vi "Read CorrectionFactors.vi"(8 "error in (no error)":errorcluster, 11 "SamplerPluginsBase in":refnum<class "SamplerPluginsBase.lvclass">) -> (0 "error out":errorcluster, 2 "CorrectionFactors":T1, 3 "SamplerPluginsBase out":refnum<class "SamplerPluginsBase.lvclass">)   [LabVIEW 2014, in "SamplerPlugins.lvlib" / "SamplerPluginsBase.lvclass"]
uses:
  SamplerPluginsBase.lvclass
  TypeDefs/CorrectionFactors.ctl
  SamplerPluginsBase.lvclass/SamplerPluginsBase.ctl
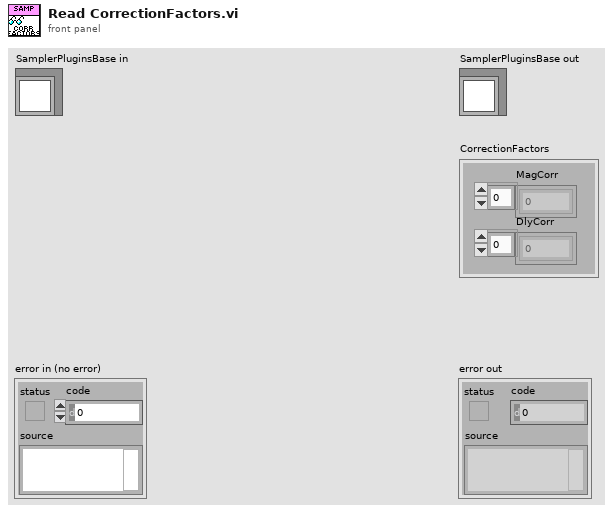
[diagram p1: front panel]
types:
  T1 = typedef "SamplerPlugins.lvlib/SamplerPluginsBase.lvclass/CorrectionFactors.ctl" = cluster{"MagCorr":dbl[], "DlyCorr":dbl[]}
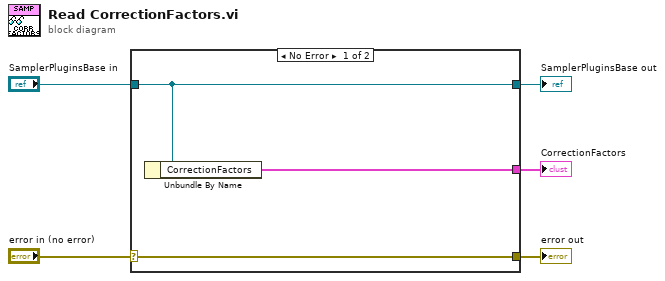
[diagram p0: block diagram]
diagram:
  n1 = case shown="No Error" "error in (no error)" {
    selector: "error in (no error)" -> [w8 w9]
    tunnel: [w8 w9] -> w4
    tunnel: [w7 w10] -> w2
    tunnel: "SamplerPluginsBase in" -> [w7 w10]
    tunnel: [w6 _] -> w1
    frame No Error {
      n2 = Unbundle By Name(w7) -> ("CorrectionFactors"=w6:T1)
    }
    frame Error {
    }
  }
  "error out" <- w4
  "SamplerPluginsBase out" <- w2
  "CorrectionFactors" <- w1
